vi "Abort.vi"(8 "error in (no error)":errorcluster, 11 "CS++Scope":refnum<class "CS++Scope.lvclass">) -> (0 "error out":errorcluster, 3 "CS++Scope out":refnum<class "CS++Scope.lvclass">)   [LabVIEW 2013, in "CS++Scope.lvlib" / "CS++Scope.lvclass"]
doc: "This VI aborts an acquisition and returns the oscilloscope to the Idle state. You initiate an acquisition with the IviScope Initiate Acquisition VIs.\n\nNotes:\n\n(1) This VI does not check the instrument status. Typically, you call this VI only in a sequence of calls to other low-level driver VIs. The sequence performs one operation. You use the low-level VIs to optimize one or more aspects of interaction with the instrument. If you want to check the instrument status, call the IviScope Error-Query VI at the conclusion of the sequence."
uses:
  CS++Scope.lvclass
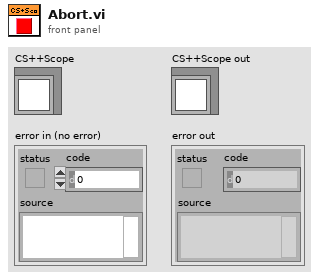
[diagram p1: front panel]
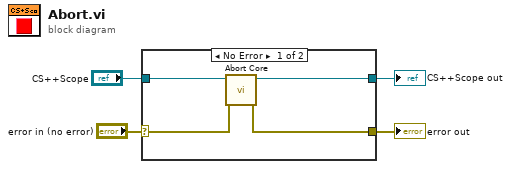
[diagram p0: block diagram]
diagram:
  n1 = case shown="No Error" "error in (no error)" {
    selector: "error in (no error)" -> [w6 w10]
    tunnel: [w5 w10] -> w3
    tunnel: [w7 w9] -> w2
    tunnel: "CS++Scope" -> [w8 w9]
    frame No Error {
      n2 = call-dynamic "Abort Core.vi"("error in (no error)"=w6, "CS++Scope"=w8) -> ("error out"=w5:errorcluster, "CS++Scope out"=w7:refnum<class "CS++Scope.lvclass">)  [unwired: 8 in]
    }
    frame Error {
    }
  }
  "error out" <- w3
  "CS++Scope out" <- w2
